vi "Send To Receivers.vi"(8 "error in (no error)":errorcluster, 9 "priority":T1, 10 "Message":refnum<class "Message.lvclass">, 11 "Pub Sub Message Channel in":refnum<class "Pub Sub Message Channel.lvclass">) -> (0 "error out":errorcluster)   [LabVIEW 2020, in "Actor Pub Sub Channels.lvlib" / "Pub Sub Message Channel.lvclass"]
uses:
  Pub Sub Message Channel.lvclass
  <vilib>/ActorFramework/Message/Message.lvclass
  <vilib>/ActorFramework/Message Dequeuer/Dequeue Priority.ctl
  Pub Sub Message Channel.lvclass/Pub Sub Message Channel.ctl
  <vilib>/ActorFramework/Self-Addressed Msg/Self-Addressed Msg.lvclass/Self-Addressed Msg.ctl
  <vilib>/ActorFramework/Message Enqueuer/Message Enqueuer.lvclass
  <vilib>/ActorFramework/Self-Addressed Msg/Self-Addressed Msg.lvclass
  <vilib>/ActorFramework/Message Dequeuer/Message Dequeuer.lvclass
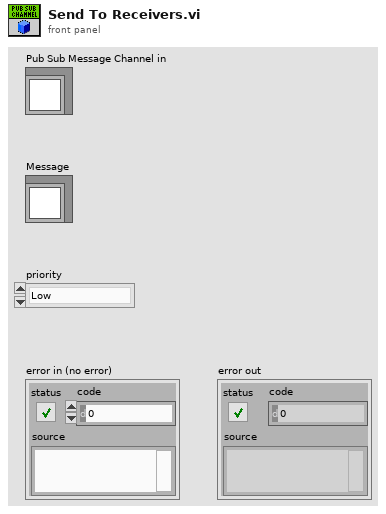
[diagram p1: front panel]
types:
  T1 = typedef "Actor Framework.lvlib/Message Dequeuer.lvclass/Dequeue Priority.ctl" = enum16{"Low", "Normal", "High", "Critical"}
  T2 = map{refnum<class "Message Enqueuer.lvclass">, cluster{"Name":string, "Included (All)":refnum<class "Message.lvclass">[], "Excluded (None)":refnum<class "Message.lvclass">[]}}
  T3 = cluster{"Name":string, "Included (All)":refnum<class "Message.lvclass">[], "Excluded (None)":refnum<class "Message.lvclass">[]}
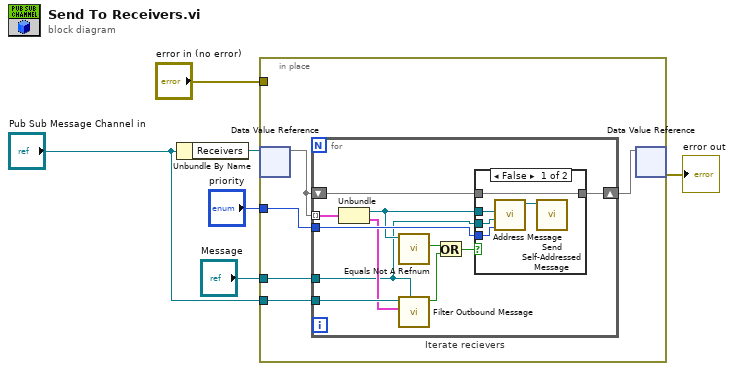
[diagram p0: block diagram]
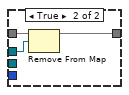
[diagram p2: hidden frame]
diagram:
  n1 = Unbundle By Name("Pub Sub Message Channel in") -> ("Receivers"=w4:refnum<data-value>)
  n2 = in-place {
    in-place-border: "Message" -> [w11]
    in-place-border: "priority" -> [w10]
    in-place-border: "error in (no error)" -> [_]
    in-place-border: "Pub Sub Message Channel in" -> [w7]
    n3 = in-place-dvr #1(w4) -> (w9:T2)  [unwired: 1 out]
    n4 = for "Iterate recievers" {
      tunnel: w9 -> [w22] mode=indexing
      tunnel: w11 -> [w14]
      tunnel: w10 -> [w18]
      shift-right: [w20] -> w8
      shift-left: w9 -> [w21]
      tunnel: w7 -> [w16]
      n5 = Unbundle(w22) -> ("Message Enqueuer"=w17:refnum<class "Message Enqueuer.lvclass">, w15:T3)
      n6 = call <vilib>:"Equals Not A Refnum.vi"("Message Enqueuer"=w17) -> ("Not a refnum?"=w19:bool)  [unwired: 10 in]
      n7 = call "Filter Outbound Message.vi"("Message"=w14, "Receiver Info"=w15, "Pub Sub Message Channel in"=w16) -> ("Drop Message"=w12:bool)  [unwired: 8 in]
      n8 = Or(x=w19, y=w12) -> (x .or. y?=w13:bool)
      n9 = case shown="False" w13 {
        tunnel: w21 -> [w23 w30]
        tunnel: [w23 w29] -> w20
        tunnel: w17 -> [w24 w28]
        tunnel: w18 -> [w27 _]
        tunnel: w14 -> [w26 _]
        frame False {
          n10 = call <vilib>:"Address Message.vi"("Message Priority (Normal)"=w27, "Message"=w26, "Destination"=w24) -> ("Self-Addressed Message"=w25:refnum<class "Self-Addressed Msg.lvclass">)  [unwired: 8 in]
          n11 = call-dynamic "Send Self-Addressed Message.vi"("Self-Addressed Message in"=w25) -> ()  [unwired: 9 in, 2 out]
        }
        frame True {
          n12 = Remove From Map(10:w28, 11:w30) -> (3:w29:T2)  [unwired: 2 out]
        }
      }
    }
    n13 = in-place-dvr #1(w8) -> (→"error out":errorcluster)  [unwired: 1 out]
  }
